vi "Set Device Baud Rate.vi"(8 "Error In":errorcluster, 10 "Baud Rate":u32, 11 "LINX Device Config":T1) -> (0 "Error Out":errorcluster, 2 "Baud Rate":u32, 3 "LINX Device Config":T1)   [LabVIEW 2014, in "LMH-LINX.lvlib" / "Device.lvlib"]
uses:
  <vilib>/MakerHub/LINX/Private/Device/Device.lvlib
  <vilib>/MakerHub/LINX/Private/Device/Type Defs/LINX Device Config.ctl
  <vilib>/MakerHub/LINX/Private/Type Defs/Interface.ctl
  <vilib>/MakerHub/LINX/Private/Device/Type Defs/TCP Config.ctl
  <vilib>/MakerHub/LINX/Private/Device/Type Defs/Channels.ctl
  <vilib>/MakerHub/LINX/Private/Type Defs/Error Type.ctl
  <vilib>/MakerHub/LINX/LMH-LINX.lvlib
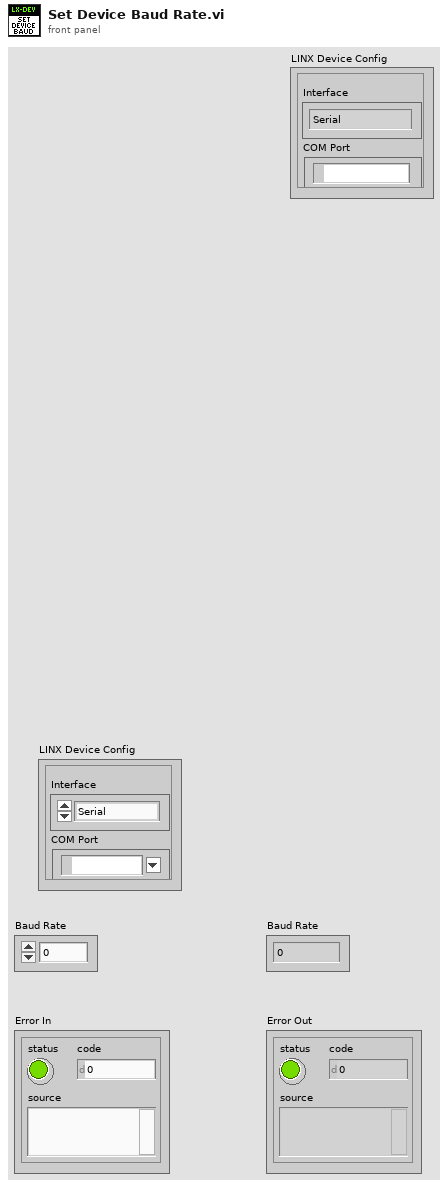
[diagram p1: front panel]
types:
  T1 = typedef "LMH-LINX.lvlib/Device.lvlib/LINX Device Config.ctl" = cluster{"Interface":T2, "COM Port":refnum<visa-resource-name>, "TCP Configuration":T3, "Device Family":u8, "Device ID":u8, "Device Name":string, "TCP Ref":refnum<k5>, "Channels":T4}
  T2 = typedef "LMH-LINX.lvlib/Interface.ctl" = enum16{"Serial", "TCP"}
  T3 = typedef "LMH-LINX.lvlib/Device.lvlib/TCP Config.ctl" = cluster{"IP Address":string, "Port":u16}
  T4 = typedef "LMH-LINX.lvlib/Channels.ctl" = cluster{"DI":u8[], "DO":u8[], "AI":u8[], "AO":u8[], "PWM":u8[], "QE":u8[], "UART":u8[], "I2C 2":u8[], "SPI":u8[], "CAN":u8[], "Servo":u8[], "AI Ref (V)":dbl, "AI Resolution (Bits)":u8, "AO Ref (V)":dbl, "AO Resolution (Bits)":u8}
  T5 = typedef "LMH-LINX.lvlib/Error Type.ctl" = enum16{"Unknown", "Timeout", "Corrupt Return Packet", "Unable To Connect", "Command Not Supported", "Channel DNE", "Invalid COM Config", "Firmware Version Mismatch", "myRIO Support", "CMD Specific Error", "Local IO Not Supported"}
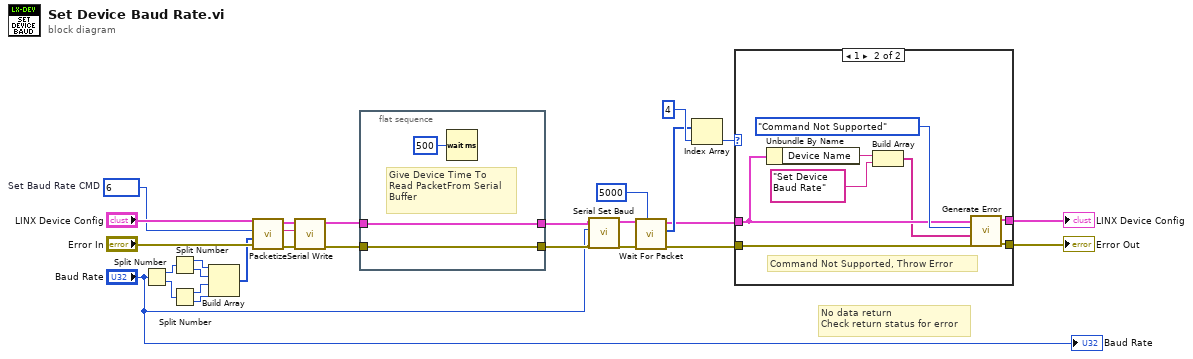
[diagram p0: block diagram]
diagram:
  w15 = u16 6  # Set Baud Rate CMD
  # "No data return\nCheck return status for error"
  n1 = Split Number(x="Baud Rate") -> (hi(x)=w24:u16, lo(x)=w25:u16)
  n2 = Split Number(x=w24) -> (hi(x)=w23:u8, lo(x)=w22:u8)
  n3 = Split Number(x=w25) -> (hi(x)=w21:u8, lo(x)=w20:u8)
  n4 = Build Array(w23, w22, w21, w20) -> (w14:u8[])
  n5 = call <vilib>:"Packetize.vi"("Error In"="Error In", "ARGS"=w14, "CMD"=w15, "LINX Device Config"="LINX Device Config") -> ("Error Out"=w18:errorcluster, "Packet"=w8:string, "LINX Decice Config"=w19:T1)  [unwired: 5 in]
  n6 = call <vilib>:"Serial Write.vi"("Error In"=w18, "Data"=w8, "LINX Device Config"=w19) -> ("Error Out"=w7:errorcluster, "LINX Device Config"=w6:T1)  [unwired: 7 in]
  n7 = flat-sequence {
    tunnel: [w30] -> w3
    tunnel: w7 -> [w30]
    tunnel: w6 -> [w29]
    tunnel: [w29] -> w2
    frame #0 {
      # "Give Device Time To \nRead PacketFrom Serial \nBuffer"
      n8 = Wait (ms)(milliseconds to wait=u32 500) -> ()  [unwired: 1 out]
    }
  }
  n9 = call <vilib>:"Serial Set Baud.vi"("Error In"=w3, "Baud Rate"="Baud Rate", "LINX Device Config"=w2) -> ("Error Out"=w4:errorcluster, "LINX Device Config"=w5:T1)  [unwired: 7 in]
  n10 = call <vilib>:"Wait For Packet.vi"("Timeout (100 ms)"=u32 5000, "Error In"=w4, "LINX Device Config"=w5) -> ("Error Out"=w11:errorcluster, "Packet"=w12:u8[], "LINX Device Config"=w10:T1)  [unwired: 6 in]
  n11 = Index Array(array=w12, index=4) -> (element=w13:u8)
  n12 = case shown="1" w13 {
    tunnel: [w33 w40] -> w27
    tunnel: [w32 w41] -> w26
    tunnel: w11 -> [w32 w38]
    tunnel: w10 -> [w33 w35]
    frame 0, Default {
      # "Read Device Reboot Delay"
      # "Status OK"
    }
    frame 1 {
      # "Command Not Supported, Throw Error"
      n13 = Unbundle By Name(w35) -> ("Device Name"=w37:string)
      n14 = Build Array(w37, "Set Device Baud Rate") -> (w34:string[])
      n15 = call <vilib>:"Generate Error.vi"("Error In"=w38, "Arguments"=w34, "Error Type"=Error_Type."Command Not Supported", "LINX Device Config"=w35) -> ("Error Out"=w41:errorcluster, "Dup LINX Device Config"=w40:T1)  [unwired: 6 in]
    }
  }
  "Error Out" <- w26
  "LINX Device Config" <- w27
  "Baud Rate" <- "Baud Rate"
